vi "Calibrate VNA.vi"(8 "error in (no error)":errorcluster, 9 "Cal kit type":enum16{"E-CAL", "Mechanical"}(ring), 10 "Calibration mode":enum16{"1 Port", "2  Port", "3 Port", "4 Port"}(ring), 11 "VNA-ENA in":refnum<class "VNA-ENA.lvclass">) -> (0 "error out":errorcluster, 3 "VNA-ENA out":refnum<class "VNA-ENA.lvclass">)   [LabVIEW 2020, in "VNA-ENA.lvclass"]
uses:
  VNA-ENA.lvclass
  Vector Network Analyzer.lvclass
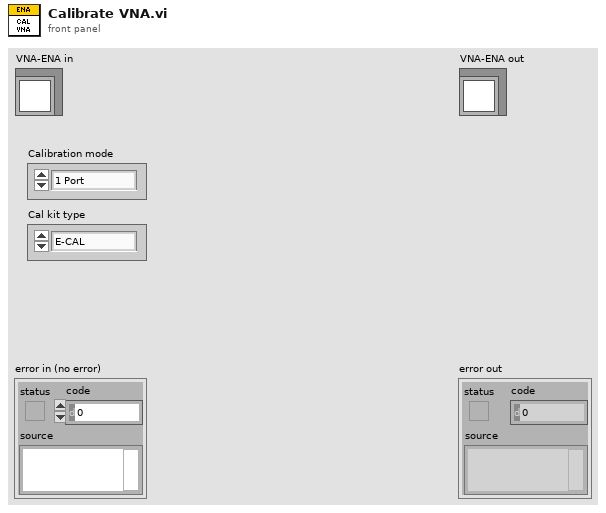
[diagram p1: front panel]
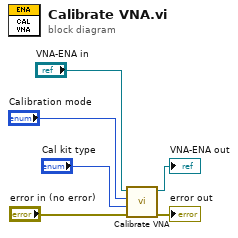
[diagram p0: block diagram]
diagram:
  n1 = call-parent "Calibrate VNA.vi"("error in (no error)"="error in (no error)", "Cal kit type"="Cal kit type", "Calibration mode"="Calibration mode", "Vector Network Analyzer in"="VNA-ENA in") -> ("error out"=→"error out":errorcluster, "Vector Network Analyzer out"=→"VNA-ENA out":refnum<class "VNA-ENA.lvclass">)  [unwired: 6 in]
